vi "DIO Valve Set.vi"(10 "current time":timestamp, 11 "State in":T1={"State"=enum."Measuring", "Start Time"=timestamp(0 s since 1904-01-01), "Current Time"=timestamp(0 s since 1904-01-01), "First Iteration"=FALSE, "Data"={"D-O State"=enum."Off"}, "Process Name"="", "Output Error"=FALSE, "Log Started"=FALSE, "Cycle Period"=0.0, "Configuration"={"Valve Settings"={"D-O Settings"={"DAQmx Task Name"="", "Output Channel"=0, "Output Channel Names"=[]}, "VICI Electronic Actuator"={"VISA resource name"="", "Mode"=enum."Two Positions With Stops", "Simulated"=FALSE}}, "Valve Type"=enum."Digital Output Valve", "Time On (Sec)"=0.0, "Time Off (Sec)"=0.0, "Run?"=FALSE}} {"Configuration"."Valve Settings"."D-O Settings"."Output Channel" items=["Choose a Channel"]}) -> (1 "time":timestamp, 2 "Numeric":i32, 3 "State out":T1={"State"=enum."Measuring", "Start Time"=timestamp(0 s since 1904-01-01), "Current Time"=timestamp(0 s since 1904-01-01), "First Iteration"=FALSE, "Data"={"D-O State"=enum."Off"}, "Process Name"="", "Output Error"=FALSE, "Log Started"=FALSE, "Cycle Period"=0.0, "Configuration"={"Valve Settings"={"D-O Settings"={"DAQmx Task Name"="", "Output Channel"=0, "Output Channel Names"=[]}, "VICI Electronic Actuator"={"VISA resource name"="", "Mode"=enum."Two Positions With Stops", "Simulated"=FALSE}}, "Valve Type"=enum."Digital Output Valve", "Time On (Sec)"=0.0, "Time Off (Sec)"=0.0, "Run?"=FALSE}} {"Configuration"."Valve Settings"."D-O Settings"."Output Channel" items=["Choose a Channel"]})   [LabVIEW 2018, in "D-O Module.lvlib" / "D-O Module Engine.lvlib"]
uses:
  Measure Instrument/D-O Module Engine.lvlib
  Measure Instrument/State Cluster.ctl
  Measure Instrument/State Enum.ctl
  Valve Clusters.ctl
  D-O Module Settings Cluster.ctl
  D-O Device Settings Cluster.ctl
  VICI Electronic Actuator/VICI Electronic Actuator Settings.ctl
  Tag VIs/Tag FGV Operation Enum.ctl
  Shared Variables/Dynamic Shared Variables.lvlib
  VICI Electronic Actuator.lvlib
  D-O Module.lvlib
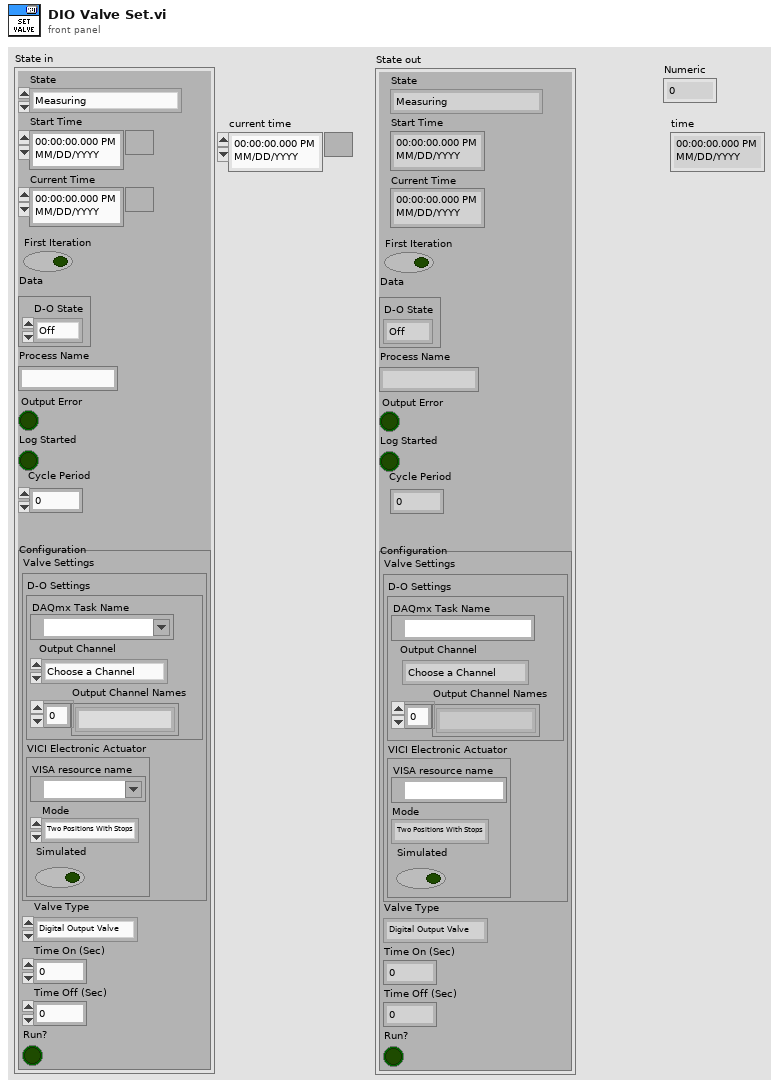
[diagram p1: front panel]
types:
  T1 = typedef "D-O Module.lvlib/D-O Module Engine.lvlib/State Cluster.ctl" = cluster{"State":T2, "Start Time":timestamp, "Current Time":timestamp, "First Iteration":bool, "Data":cluster{"D-O State":enum16{"Off", "On", "Not Initialized"}}, "Process Name":string, "Output Error":bool, "Log Started":bool, "Cycle Period":dbl, "Configuration":T3}
  T2 = typedef "D-O Module.lvlib/D-O Module Engine.lvlib/State Enum.ctl" = enum16{"Measuring", "Idle", "Paused"}
  T3 = typedef "D-O Module.lvlib/Valve Clusters.ctl" = cluster{"Valve Settings":T4, "Valve Type":enum16{"Default", "Digital Output Valve", "VICI Electronic Actuator"}, "Time On (Sec)":dbl, "Time Off (Sec)":dbl, "Run?":bool}
  T4 = typedef "D-O Module.lvlib/D-O Module Settings Cluster.ctl" = cluster{"D-O Settings":T5, "VICI Electronic Actuator":T6}
  T5 = typedef "D-O Module.lvlib/D-O Device Settings Cluster.ctl" = cluster{"DAQmx Task Name":refnum<k21>, "Output Channel":u16, "Output Channel Names":string[]}
  T6 = typedef "VICI Electronic Actuator.lvlib/VICI Electronic Actuator Settings.ctl" = cluster{"VISA resource name":refnum<visa-resource-name>, "Mode":enum16{"Two Positions With Stops", "Two Positions Without Stops", "Mutiposition"}, "Simulated":bool}
  T7 = enum16{"Default", "Digital Output Valve", "VICI Electronic Actuator"}
  T8 = typedef "Tag FGV Operation Enum.ctl" = enum16{"Init", "Set Notification Queue", "Create Tag", "Commit", "Write Tag (Numeric)", "Write Tag (Boolean)", "Read All Tags", "Read One Tag", "Delete Tag Category", "Set Alarm Parameters (Numeric)", "Set Alarm Parameters (Boolean)", "Enable All Alarms", "Disable All Alarms", "Delete All Tags", "Read Alarms", "Ack Alarm", "Read Alarm Parameters (Numeric)", "Read Alarm Parameters (Boolean)"}
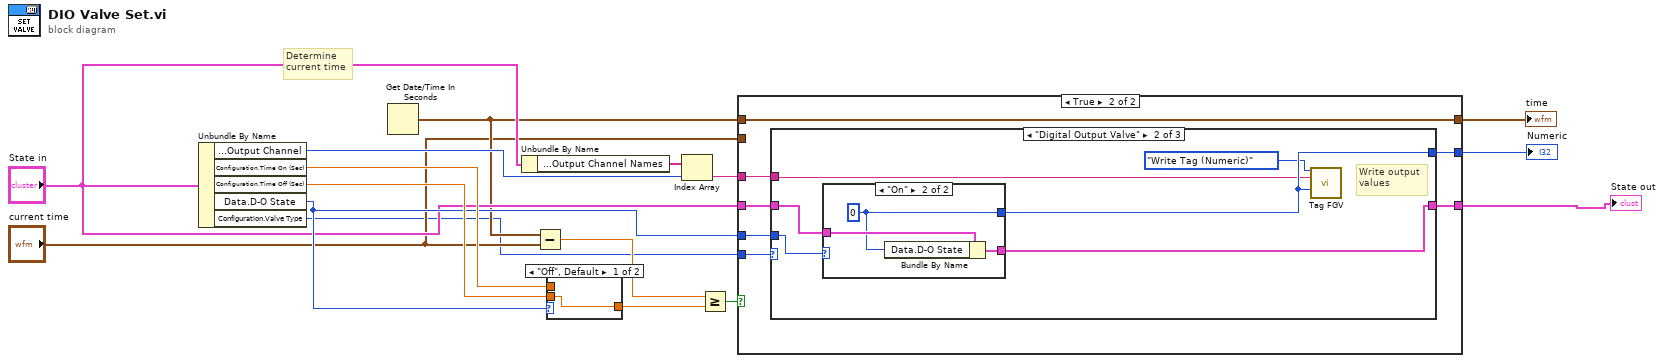
[diagram p0: block diagram]
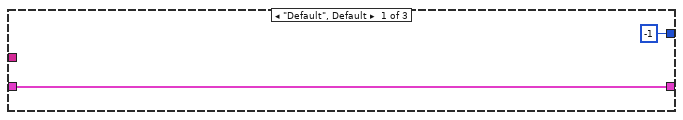
[diagram p4: hidden frame]
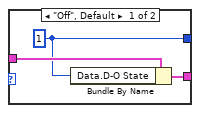
[diagram p5: hidden frame]
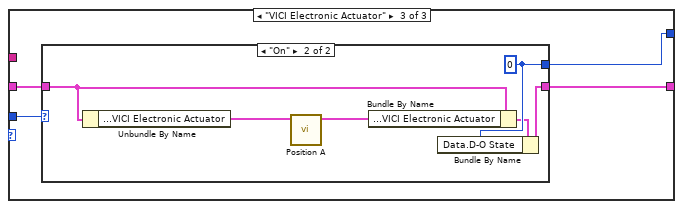
[diagram p6: hidden frame]
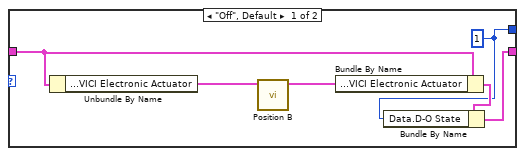
[diagram p7: hidden frame]
diagram:
  # "Determine\ncurrent time"
  n1 = Unbundle By Name("State in") -> ("Configuration.Valve Settings.D-O Settings.Output Channel"=w11:u16, "Configuration.Time On (Sec)"=w14:dbl, "Configuration.Time Off (Sec)"=w15:dbl, "Data.D-O State"=w12:enum16{"Off", "On", "Not Initialized"}, "Configuration.Valve Type"=w4:T7)
  n2 = Get Date/Time In Seconds() -> (seconds since 1Jan1904=w7:timestamp)
  n3 = Unbundle By Name("State in") -> ("Configuration.Valve Settings.D-O Settings.Output Channel Names"=w10:string[])
  n4 = Subtract(x=w7, y="current time") -> (x-y=w8:dbl)
  n5 = case shown="\"Off\", Default" w12 {
    tunnel: [w17 w18] -> w16
    tunnel: w15 -> [w17 _]
    tunnel: w14 -> [_ w18]
    frame "Off", Default {
    }
    frame "On" {
    }
  }
  n6 = Index Array(array=w10, index=w11) -> (element=w3:string)
  n7 = Greater Or Equal?(x=w8, y=w16) -> (x >= y?=w13:bool)
  n8 = case shown="True" w13 {
    tunnel: [w21 w28] -> w2
    tunnel: "State in" -> [w20 w26]
    tunnel: [w20 w27] -> w1
    tunnel: w12 -> [w21 w25]
    tunnel: w7 -> [_ w24]
    tunnel: "current time" -> [w19 _]
    tunnel: [w19 w24] -> w5
    tunnel: w4 -> [_ w23]
    tunnel: w3 -> [_ w22]
    frame False {
    }
    frame True {
      n9 = case shown="\"Digital Output Valve\"" w23 {
        tunnel: [-1 w33 w44] -> w28
        tunnel: [w30 w36 w45] -> w27
        tunnel: w26 -> [w30 w35 w46]
        tunnel: w25 -> [_ w34 w43]
        tunnel: w22 -> [_ w31 _]
        frame "Default", Default {
        }
        frame "Digital Output Valve" {
          # "Write output\nvalues"
          n10 = case shown="\"On\"" w34 {
            tunnel: w35 -> [w39 w42]
            tunnel: [w38 w40] -> w36
            tunnel: [w37 w41] -> w33
            frame "Off", Default {
              w37 = 1
              n11 = Bundle By Name(cluster=w39, "Data.D-O State"=w37) -> (w38:T1)
            }
            frame "On" {
              w41 = 0
              n12 = Bundle By Name(cluster=w42, "Data.D-O State"=w41) -> (w40:T1)
            }
          }
          n13 = call "Tag FGV.vi"("Operation"=Tag_FGV_Operation_Enum."Write Tag (Numeric)", "Tag Name"=w31, "Data"=w33) -> ()  [unwired: 5 in, 8 out]
        }
        frame "VICI Electronic Actuator" {
          n14 = case shown="\"On\"" w43 {
            tunnel: w46 -> [w51 w58]
            tunnel: [w48 w53] -> w45
            tunnel: [w47 w55] -> w44
            frame "Off", Default {
              w47 = 1
              n15 = Unbundle By Name(w51) -> ("Configuration.Valve Settings.VICI Electronic Actuator"=w52:T6)
              n16 = call "Position B.vi"("VICI Electronic Actuator"=w52) -> ("VICI Electronic Actuator"=w50:T6)  [unwired: 8 in, 2 out]
              n17 = Bundle By Name(cluster=w51, "Configuration.Valve Settings.VICI Electronic Actuator"=w50) -> (w49:T1)
              n18 = Bundle By Name(cluster=w49, "Data.D-O State"=w47) -> (w48:T1)
            }
            frame "On" {
              w55 = 0
              n19 = Unbundle By Name(w58) -> ("Configuration.Valve Settings.VICI Electronic Actuator"=w57:T6)
              n20 = call "Position A.vi"("VICI Electronic Actuator"=w57) -> ("VICI Electronic Actuator"=w56:T6)  [unwired: 7 in, 3 out]
              n21 = Bundle By Name(cluster=w58, "Configuration.Valve Settings.VICI Electronic Actuator"=w56) -> (w54:T1)
              n22 = Bundle By Name(cluster=w54, "Data.D-O State"=w55) -> (w53:T1)
            }
          }
        }
      }
    }
  }
  "Numeric" <- w2
  "State out" <- w1
  "time" <- w5
